vi "Get Key Info.vi"(8 "error in (no error)":errorcluster, 11 "CngKey in":refnum<k24>) -> (0 "error out":errorcluster, 2 "Key Information":T1, 3 "CngKey out":refnum<k24>)   [LabVIEW 2021, in "dotNET Crypto Key Management.lvlib"]
uses:
  dotNET Crypto Key Management.lvlib
  System.Core
  CNG Key Info.ctl
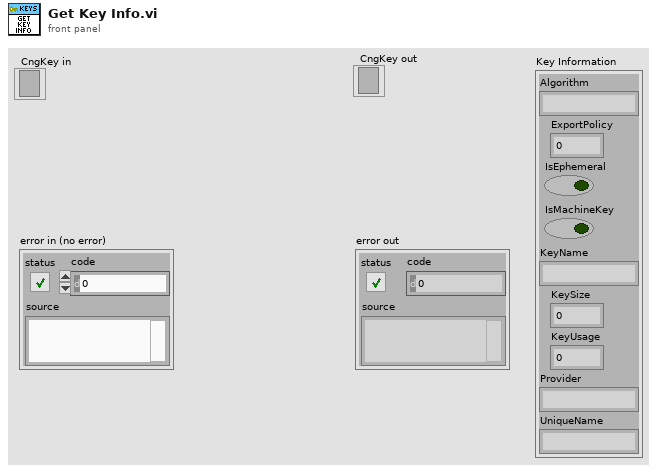
[diagram p1: front panel]
types:
  T1 = typedef "dotNET Crypto Key Management.lvlib/CNG Key Info.ctl" = cluster{"Algorithm":string, "ExportPolicy":i32, "IsEphemeral":bool, "IsMachineKey":bool, "KeyName":string, "KeySize":i32, "KeyUsage":i32, "Provider":string, "UniqueName":string}
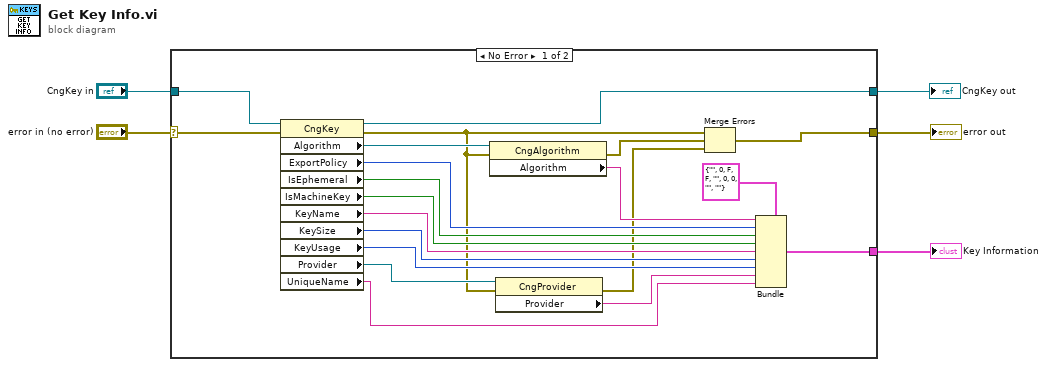
[diagram p0: block diagram]
diagram:
  n1 = case shown="No Error" "error in (no error)" {
    selector: "error in (no error)" -> [w10 w27]
    tunnel: "CngKey in" -> [w25 w26]
    tunnel: [w24 w26] -> w4
    tunnel: [w11 _] -> w3
    tunnel: [w6 w27] -> w1
    frame No Error {
      n2 = property class="CngKey"(reference=w25, error in=w10) -> (reference out=w24:refnum<k24>, error out=w9:errorcluster, "Algorithm"=w23:refnum<k24>, "ExportPolicy"=w20:i32, "IsEphemeral"=w19:bool, "IsMachineKey"=w18:bool, "KeyName"=w17:string, "KeySize"=w16:i32, "KeyUsage"=w15:i32, "Provider"=w22:refnum<k24>, "UniqueName"=w13:string)
      n3 = property class="CngAlgorithm"(reference=w23, error in=w9) -> (error out=w8:errorcluster, "Algorithm"=w21:string)  [unwired: 1 out]
      n4 = property class="CngProvider"(reference=w22, error in=w9) -> (error out=w7:errorcluster, "Provider"=w14:string)  [unwired: 1 out]
      n5 = Merge Errors(w9, w8, w7) -> (w6:errorcluster)
      n6 = Bundle(cluster=T1 {"Algorithm"="", "ExportPolicy"=0, "IsEphemeral"=FALSE, "IsMachineKey"=FALSE, "KeyName"="", "KeySize"=0, "KeyUsage"=0, "Provider"="", "UniqueName"=""}, "Algorithm"=w21, "ExportPolicy"=w20, "IsEphemeral"=w19, "IsMachineKey"=w18, "KeyName"=w17, "KeySize"=w16, "KeyUsage"=w15, "Provider"=w14, "UniqueName"=w13) -> (w11:T1)
    }
    frame Error {
    }
  }
  "CngKey out" <- w4
  "Key Information" <- w3
  "error out" <- w1
